vi "FromRepo.vi"(8 "error in":errorcluster, 9 "cluster":T2, 10 "repository in":refnum<class "NISE_CEF_Repository.lvclass">, 11 "cRIO in":refnum<class "cRIO.lvclass">) -> (0 "error out":errorcluster, 2 "repository out":refnum<class "NISE_CEF_Repository.lvclass">, 3 "node":T1)   [LabVIEW 2013, in "cRIO.lvclass"]
uses:
  cRIO.lvclass
  CEF_TreeControl/Repository/NISE_CEF_Repository.lvclass
  CEF_TreeControl/Node/FromRepoCluster.ctl
  CEF_TreeControl/Node/NodeRef.ctl
  CEF_TreeControl/Node/NISE_CEF_Node.lvclass
  cRIO Repo/cRIORepo.lvclass
  cRIO Repo/cRIORepo.lvclass/cRIORepo.ctl
  cRIO.lvclass/cRIO.ctl
  cRIO Repo/Read Channels.vi
  Write System Name.vi
  CEF_TreeControl/NISE_CEF_TreeControl.lvlib
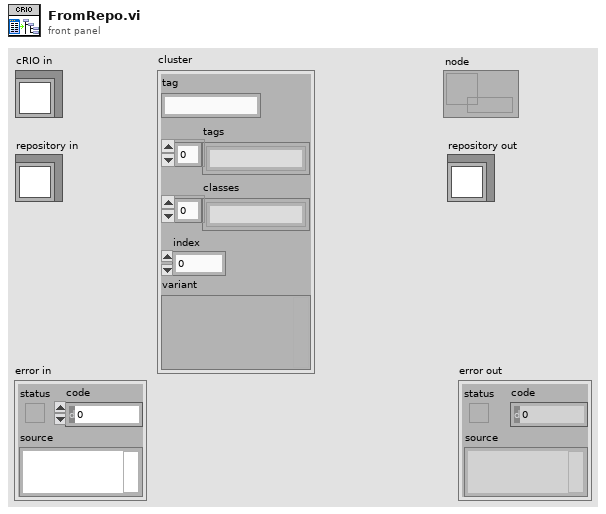
[diagram p1: front panel]
types:
  T1 = typedef "NISE_CEF_Node.lvclass/NodeRef.ctl" = refnum<data-value>
  T2 = typedef "NISE_CEF_Node.lvclass/FromRepoCluster.ctl" = cluster{"tag":string, "tags":string[], "classes":string[], "index":i32, "variant":variant}
  T3 = typedef "Channel.ctl" = cluster{"channel group":string, "channel name":string, "IO ":string, "sensor ID":string, "description":string, "system":string, "channel type":string}
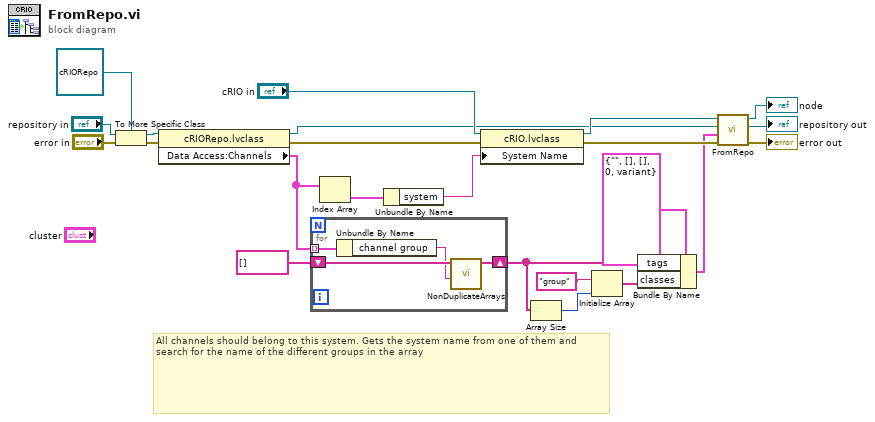
[diagram p0: block diagram]
diagram:
  # "All channels should belong to this system. Gets the system name from one of them and search for the name of the different groups in the array"
  n1 = To More Specific Class(target class=refnum<class "cRIORepo.lvclass"> refnum ("cRIO repo.lvclass"), reference="repository in", error in="error in") -> (specific class reference=w17:refnum<class "cRIORepo.lvclass">, error out=w13:errorcluster)
  n2 = property class="cRIORepo.lvclass"(reference=w17, error in=w13) -> (reference out=w16:refnum<class "cRIORepo.lvclass">, error out=w12:errorcluster, "Data Access:Channels"=w3:T3[])
  n3 = for {
    shift-right: [w25] -> w8
    shift-left: string[] [] ("array in") -> [w26]
    tunnel: w3 -> [w27] mode=indexing
    n4 = Unbundle By Name(w27) -> ("channel group"=w24:string)
    n5 = call "NonDuplicateArrays.vi"("string in"=w24, "array in"=w26) -> ("array out"=w25:string[])  [unwired: 8 in, 1 out]
  }
  n6 = Index Array(array=w3) -> (element=w2:T3)  [unwired: 1 in]
  n7 = Unbundle By Name(w2) -> ("system"=w1:string)
  n8 = property class="cRIO.lvclass"(reference="cRIO in", error in=w12, "System Name"=w1) -> (reference out=w20:refnum<class "cRIO.lvclass">, error out=w11:errorcluster)
  n9 = Array Size(array=w8) -> (size(s)=w7:i32)
  n10 = Initialize Array("group" ("System"), w7) -> (w5:string[])
  n11 = Bundle By Name(cluster=T2 {"tag"="", "tags"=[], "classes"=[], "index"=0, "variant"=variant} ("Cluster"), "tags"=w8, "classes"=w5) -> (w9:T2)
  n12 = call-parent "FromRepo.vi"("error in"=w11, "from repo cluster"=w9, "repository in"=w16, "node in"=w20) -> ("error out"=→"error out":errorcluster, "repository out"=→"repository out":refnum<class "NISE_CEF_Repository.lvclass">, "node"=→"node":T1)  [unwired: 5 in]
